vi "getTemperature.vi"(8 "error in":errorcluster) -> (0 "error out":errorcluster, 3 "Temperature":dbl)   [LabVIEW 2024]
doc: "Funkcja służy do pobierania informacji o aktualnej temperaturze w symulowanym piekarniku."
uses:
  TypeDefs/Heater_interface.ctl
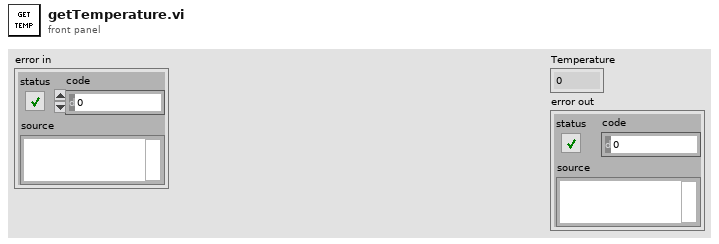
[diagram p1: front panel]
types:
  T1 = typedef "Heater_interface.ctl" = enum16{"setSpeed", "setHeaters", "getTemperature"}
  T2 = cluster{"Interface":T1, "Parameter1":variant, "Parameter2":variant}
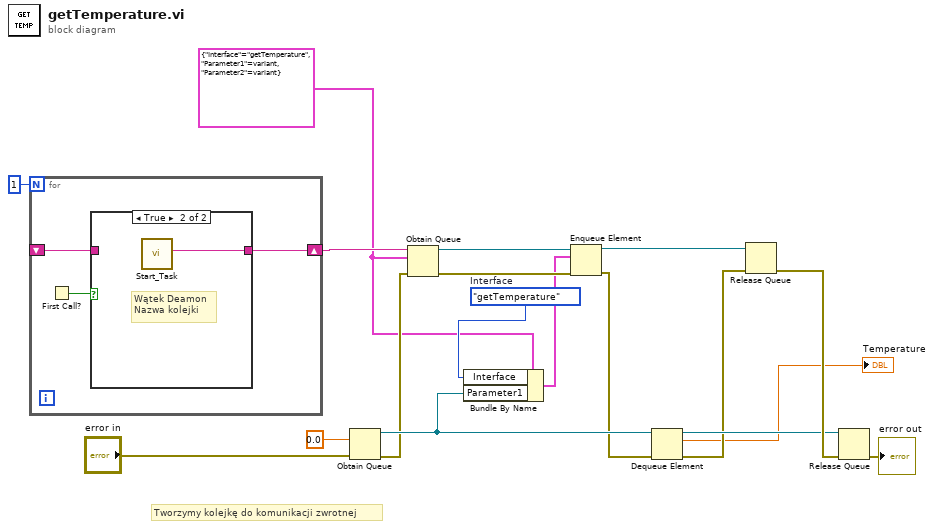
[diagram p0: block diagram]
diagram:
  w1 = T2 {"Interface"=enum."getTemperature", "Parameter1"=variant, "Parameter2"=variant}
  w2 = Heater_interface."getTemperature"  # Interface
  # "Tworzymy kolejkę do komunikacji zwrotnej"
  n1 = for {
    N: 1 -> [_]
    shift-right: [w20] -> w17
    shift-left: _ -> [w19]
    n2 = First Call?() -> (First Call?: T/F=w21:bool)
    n3 = case shown="True" w21 {
      tunnel: [w22 w23] -> w20
      tunnel: w19 -> [w22 _]
      frame False {
      }
      frame True {
        # "Wątek Deamon\nNazwa kolejki"
        n4 = call "Start_Task.vi"() -> ("QueueName"=w23:string)  [unwired: 11 in]
      }
    }
  }
  n5 = Obtain Queue(element data type=0.0, error in (no error)="error in") -> (queue out=w10:refnum<queue>, error out=w4:errorcluster)  [unwired: 3 in, 1 out]
  n6 = Obtain Queue(name (unnamed)=w17, element data type=w1, error in (no error)=w4) -> (queue out=w16:refnum<queue>, error out=w15:errorcluster)  [unwired: 2 in, 1 out]
  n7 = Bundle By Name(cluster=w1, "Interface"=w2, "Parameter1"=w10) -> (w14:T2)
  n8 = Enqueue Element(queue=w16, element=w14, error in (no error)=w15) -> (queue out=w13:refnum<queue>, error out=w8:errorcluster)  [unwired: 1 in, 1 out]
  n9 = Dequeue Element(queue=w10, error in (no error)=w8) -> (queue out=w9:refnum<queue>, element=→"Temperature":dbl, error out=w7:errorcluster)  [unwired: 1 in, 1 out]
  n10 = Release Queue(queue=w13, error in (no error)=w7) -> (error out=w11:errorcluster)  [unwired: 1 in, 2 out]
  n11 = Release Queue(queue=w9, error in (no error)=w11) -> (error out=→"error out":errorcluster)  [unwired: 1 in, 2 out]
